vi "TestTreeToRepo.vi"() -> (2 "summary":T1[](array[typedef]))   [LabVIEW 2025]
uses:
  Trunk/ProjectTemplates/Source/Configuration Editor Framework/Classes/cRIO/cRIO.lvclass
  Trunk/ProjectTemplates/Source/Configuration Editor Framework/Classes/Group/Group.lvclass
  Trunk/ProjectTemplates/Source/Configuration Editor Framework/Classes/Voltage/Voltage.lvclass
  NISE_CEF_Tests.lvlib
  Trunk/ProjectTemplates/Source/Configuration Editor Framework/Classes/cRIO Repo/cRIORepo.lvclass
  Trunk/Configuration Framework/Node/Summary.ctl
  Controls/IDs.ctl
panel:
  out "summary 2":T1[](array[typedef])
  out "error out":errorcluster
  out "Ids":T2
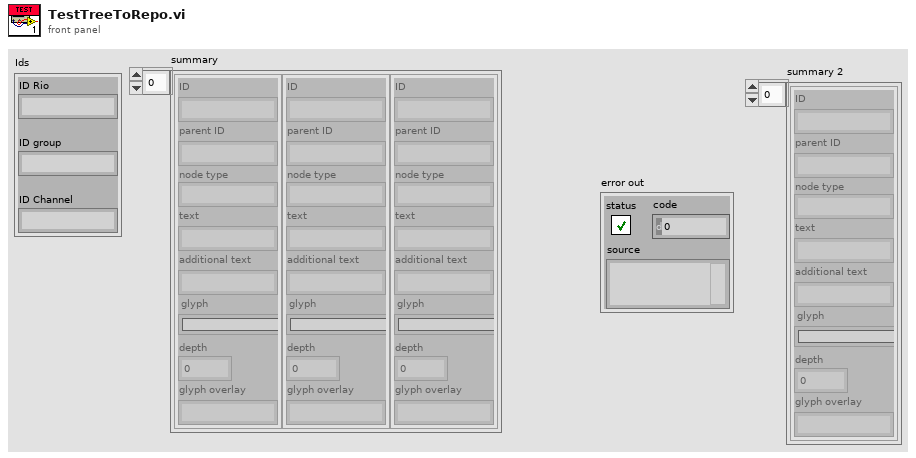
[diagram p1: front panel]
types:
  T1 = typedef "NISE_CEF_Node.lvclass/Summary.ctl" = cluster{"ID":string, "parent ID":string, "node type":string, "text":string, "additional text":string, "glyph":string, "depth":i32, "glyph overlay":string}
  T2 = typedef "NISE_CEF_Tests.lvlib/IDs.ctl" = cluster{"ID Channel":string, "ID Rio":string, "ID group":string}
  T3 = typedef "NISE_CEF_Node.lvclass/NodeRef.ctl" = refnum<data-value>
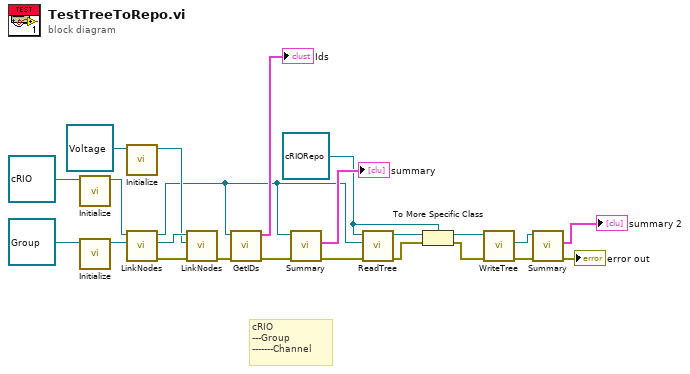
[diagram p0: block diagram]
diagram:
  w3 = refnum<class "cRIORepo.lvclass"> refnum ("cRIORepo.lvclass")
  # "cRIO\n---Group\n-------Channel"
  n1 = call-dynamic "Initialize.vi"("cRIO in"=refnum<class "cRIO.lvclass"> refnum ("cRIO.lvclass")) -> ("data value reference"=w20:T3)  [unwired: 8 in, 2 out]
  n2 = call-dynamic "Initialize.vi"("group in"=refnum<class "Group.lvclass"> refnum ("Group.lvclass")) -> ("data value reference"=w19:T3)  [unwired: 8 in, 2 out]
  n3 = call-dynamic "Initialize.vi"("voltage in"=refnum<class "Voltage.lvclass"> refnum ("Voltage.lvclass")) -> ("data value reference"=w17:T3)  [unwired: 8 in, 2 out]
  n4 = call "LinkNodes.vi"("child in"=w19, "parent in"=w20) -> ("error out"=w15:errorcluster, "child out"=w18:T3, "parent out"=w10:T3)  [unwired: 7 in]
  n5 = call "LinkNodes.vi"("error in"=w15, "child in"=w17, "parent in"=w18) -> ("error out"=w14:errorcluster)  [unwired: 6 in, 2 out]
  n6 = call "GetIDs.vi"("error in"=w14, "data value reference in"=w10) -> ("error out"=w13:errorcluster, "IDs"=→"Ids":T2)  [unwired: 6 in, 2 out]
  n7 = call "Summary.vi"("error in"=w13, "node self ref"=w10) -> ("error out"=w11:errorcluster, "summary"=→"summary":T1[])  [unwired: 8 in]
  n8 = call-dynamic "ReadTree.vi"("error in"=w11, "root"=w10, "cRIO repo in"=w3) -> ("error out"=w2:errorcluster, "repository out"=w9:refnum<class "NISE_CEF_Repository.lvclass">)  [unwired: 7 in]
  n9 = To More Specific Class(target class=w3, reference=w9, error in=w2) -> (specific class reference=w4:refnum<class "cRIORepo.lvclass">, error out=w1:errorcluster)
  n10 = call-dynamic "WriteTree.vi"("error in"=w1, "cRIO repo in"=w4) -> ("error out"=w8:errorcluster, "root"=w7:T3)  [unwired: 7 in, 1 out]
  n11 = call "Summary.vi"("error in"=w8, "node self ref"=w7) -> ("error out"=→"error out":errorcluster, "summary"=→"summary 2":T1[])  [unwired: 8 in]
